vi "GT Set Soft Limit.vi"(7 "negative":i32, 8 "error in (no error)":errorcluster caption="错误输入（无错误）", 9 "positive":i32, 10 "axis":i16, 11 "cardNum":i16) -> (0 "error out":errorcluster caption="错误输出", 3 "function return":i16)   [LabVIEW 2020, in "gts.lvlib"]
doc: "GT_API GT_SetSoftLimit(short cardNum,short axis,long positive,long negative);"
uses:
  gts.lvlib
  dll/32bit/multi_card/gts.dll
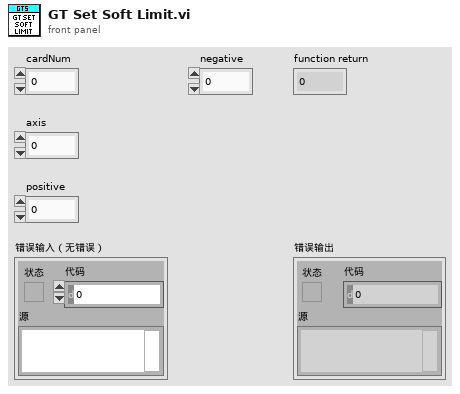
[diagram p1: front panel]
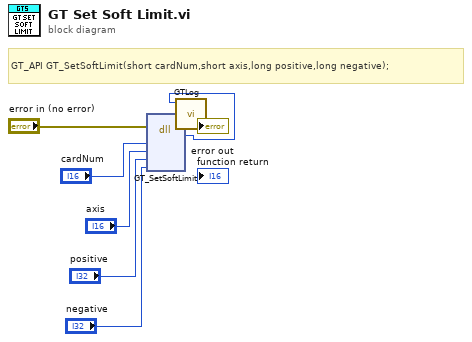
[diagram p0: block diagram]
diagram:
  # "GT_API GT_SetSoftLimit(short cardNum,short axis,long positive,long negative);"
  n1 = dll-call lib="C:/1228/dll/32bit/multi_card/gts.dll" fn="GT_SetSoftLimit"(error in="error in (no error)", "cardNum"="cardNum", "axis"="axis", "positive"="positive", "negative"="negative") -> (error out=w3:errorcluster, w1:i16)  [unwired: 6 in, 1 out]
  n2 = call "GTLog.vi"("error in (no error)"=w3, "Numeric"=w1) -> ("error out"=→"error out":errorcluster)  [unwired: 9 in]
